vi "Get systemMetrics_demo.vi"() -> ()   [LabVIEW 2012]
panel:
  out "error out":errorcluster
  out "height":u32
  out "width":u32
  in  "error in":errorcluster
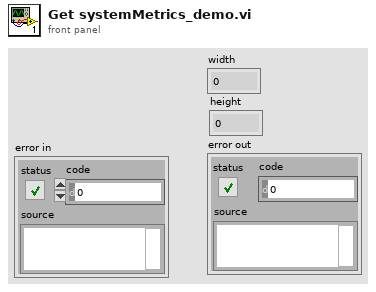
[diagram p1: front panel]
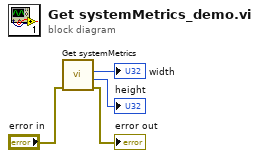
[diagram p0: block diagram]
diagram:
  n1 = call "Get systemMetrics.vi"("error in"="error in") -> ("error out"=→"error out":errorcluster, "height"=→"height":u32, "width"=→"width":u32)  [unwired: 8 in]
